vi "Release-image-references.vi"(8 "error in (no error)":errorcluster, 11 "Buffers in":refnum<class "CV-Buffers.lvclass">) -> (0 "error out":errorcluster, 3 "Buffers out":refnum<class "CV-Buffers.lvclass">)   [LabVIEW 2013, in "CameraVision.lvlib" / "CV-Buffers.lvclass"]
uses:
  CV-Buffers.lvclass
  <vilib>/vision/Image Controls.llb/IMAQ Image.ctl
  Storage-buffer-refs.ctl
  CV-Buffers.lvclass/CV-Buffers.ctl
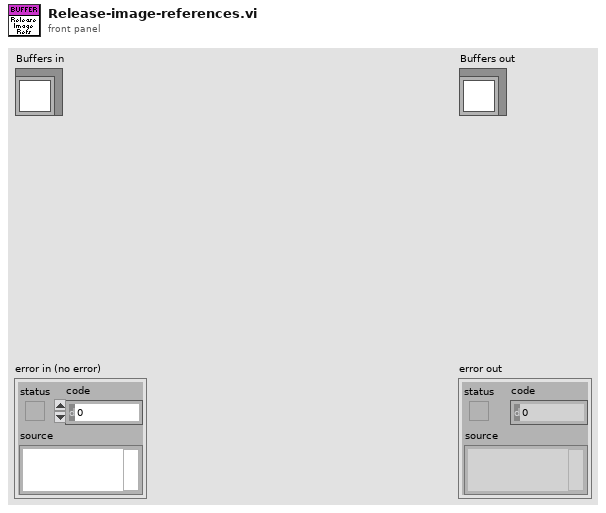
[diagram p1: front panel]
types:
  T1 = typedef "IMAQ Image.ctl" = refnum<image>
  T2 = typedef "CameraVision.lvlib/CV-Buffers.lvclass/Storage-buffer-refs.ctl" = cluster{"Raw images":T1[], "Corrected images":T1[], "Binary images":T1[]}
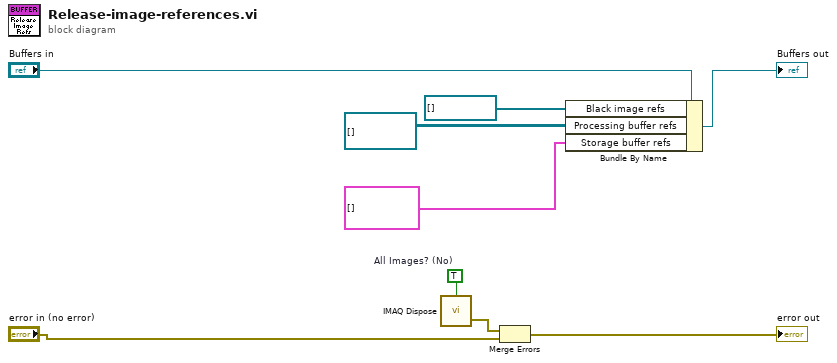
[diagram p0: block diagram]
diagram:
  w6 = TRUE  # All Images? (No)
  n1 = call "IMAQ Dispose"("All Images? (No)"=w6) -> ("error out"=w9:errorcluster)  [unwired: 5 in]
  n2 = Merge Errors(w9, "error in (no error)") -> (→"error out":errorcluster)
  n3 = Bundle By Name(cluster="Buffers in", "Black image refs"=T1[] [], "Processing buffer refs"=T1[][] [], "Storage buffer refs"=T2[] [] ("UI buffer")) -> (→"Buffers out":refnum<class "CV-Buffers.lvclass">)
